vi "Auto_Targeting.vi"(1 "Acceptable Error (deg)":dbl, 2 "Auto Targeting Enabled?":bool) -> ()   [LabVIEW 2020]
uses:
  <vilib>/Rock Robotics/WPI/ThirdParty/REV Robotics/REVLib/Typedef/Spark MAX Control Type.ctl
  <vilib>/Rock Robotics/WPI/Utilities/WPI_GetSetVariantRefNum.vi
  Global Sensor Reads.vi
  Global Shooter Speed.vi
  <vilib>/Rock Robotics/WPI/RobotDrive/WPI_RobotDriveArcadeDrive_Standard(NoSaturation).vi
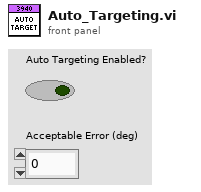
[diagram p1: front panel]
types:
  T1 = typedef "WPI_RobotDriveDevRef.ctl" = cluster{"DevStatus":errorcluster, "Motors[]":T2[], "Square Inputs":bool, "Max Output":dbl}
  T2 = typedef "WPI_MotorControlDeviceRef.ctl" = cluster{"DeviceStatus":errorcluster, "Type":T3, "PWM":cluster{"PWM Channel":T4, "DeadBand":T5}, "CAN":cluster{"Device Number":u8, "SetOutput VI Ref":variant, "GetOutput VI Ref":variant, "Enable VI Ref":variant, "Disable VI Ref":variant, "Data":variant}, "Invert":bool, "DIO PWM":cluster{"PWM \"Enable\" Channel":T4, "DIOChannel":T6, "PWM Rate":dbl}}
  T3 = typedef "WPI_MotorControlType.ctl" = enum16{"PWM", "CAN", "DIO PWM"}
  T4 = typedef "FPGA_DIOPWMChannel.ctl" = enum8{"PWM 0", "PWM 1", "PWM 2", "PWM 3", "PWM 4", "PWM 5", "PWM 6", "PWM 7", "PWM 8", "PWM 9", "PWM MXP 0", "PWM MXP 1", "PWM MXP 2", "PWM MXP 3", "PWM MXP 4", "PWM MXP 5", "PWM MXP 6", "PWM MXP 7", "PWM MXP 8", "PWM MXP 9", "Invalid"}
  T5 = typedef "WPI_PWMDeadband.ctl" = cluster{"Name":string, "maxPositivePwm":i32, "minPositivePwm":i32, "centerPwm":i32, "maxNegativePwm":i32, "minNegativePwm":i32, "angularRange":u16}
  T6 = typedef "FPGA_DIOChannel.ctl" = enum8{"DIO 0", "DIO 1", "DIO 2", "DIO 3", "DIO 4", "DIO 5", "DIO 6", "DIO 7", "DIO 8", "DIO 9", "DIO MXP 0", "DIO MXP 1", "DIO MXP 2", "DIO MXP 3", "DIO MXP 4", "DIO MXP 5", "DIO MXP 6", "DIO MXP 7", "DIO MXP 8", "DIO MXP 9", "DIO MXP 10", "DIO MXP 11", "DIO MXP 12", "DIO MXP 13", "DIO MXP 14", "DIO MXP 15", "SPI Port CS1", "SPI Port CS2", "SPI Port CS3", "SPI Port MISO", "SPI Port MOSI", "Invalid"}
  T7 = typedef "Spark MAX Control Type.ctl" = enum16{"Percent VBus", "Voltage", "Velocity", "Position", "Smart Motion", "Current", "Smart Velocity"}
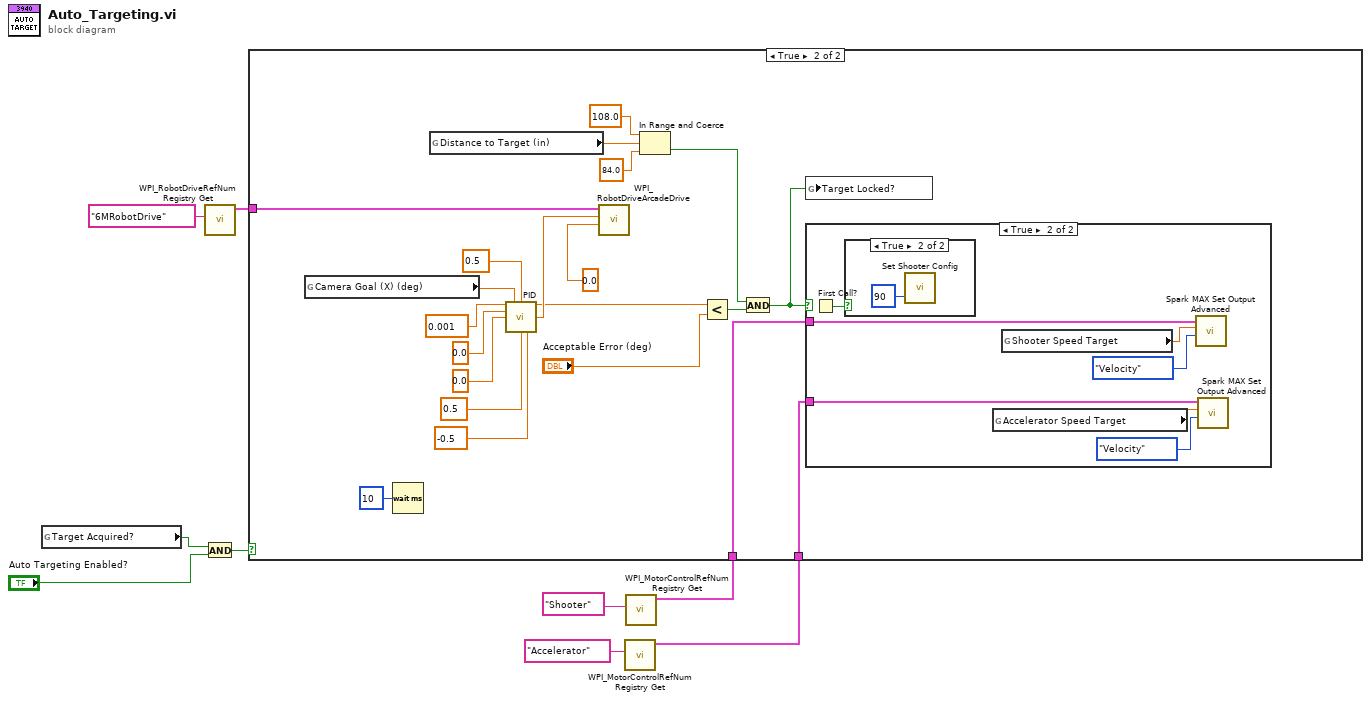
[diagram p0: block diagram]
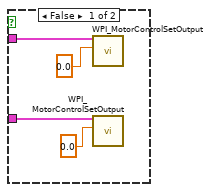
[diagram p3: hidden frame]
diagram:
  n1 = global read "Global Sensor Reads.vi" "Target Acquired?"() -> (w8:bool)
  n2 = call <vilib>:"WPI_RobotDriveRefNum Registry Get.vi"("refnum name"="6MRobotDrive") -> ("RobotDriveDevRef"=w4:T1)  [unwired: 9 in, 1 out]
  n3 = And(x=w8, y="Auto Targeting Enabled?") -> (x .and. y?=w9:bool)
  n4 = call <vilib>:"WPI_MotorControlRefNum Registry Get.vi"("refnum name"="Accelerator") -> ("MotorControlDevRef"=w2:T2)  [unwired: 9 in, 1 out]
  n5 = call <vilib>:"WPI_MotorControlRefNum Registry Get.vi"("refnum name"="Shooter") -> ("MotorControlDevRef"=w3:T2)  [unwired: 9 in, 1 out]
  n6 = case shown="True" w9 {
    tunnel: w4 -> [_ w30]
    tunnel: w3 -> [_ w29]
    tunnel: w2 -> [_ w28]
    frame False {
    }
    frame True {
      n7 = global read "Global Sensor Reads.vi" "Camera Goal (X) (deg)"() -> (w27:dbl)
      n8 = Wait (ms)(milliseconds to wait=u32 10) -> ()  [unwired: 1 out]
      n9 = global read "Global Sensor Reads.vi" "Distance to Target (in)"() -> (w15:dbl)
      n10 = call "PID.vi"("Kp"=0.001, "Process Variable"=w27, "Goal"=0.5, "Ki"=0.0, "Kd"=0.0, "Max Ouput"=0.5, "Min Output"=-0.5) -> ("Current Error"=w17:dbl, "Command"=w20:dbl)  [unwired: 6 in, 1 out]
      n11 = call-poly <vilib>:"WPI_RobotDriveArcadeDrive.vi"("Y axis value"=0.0, "X axis value"=w20, "RobotDriveDevRef"=w30) -> ()  [unwired: 6 in, 3 out]
      n12 = In Range and Coerce(upper limit=108.0, x=w15, lower limit=84.0) -> (In Range?=w11:bool)  [unwired: 1 out]
      n13 = Less?(x=w17, y="Acceptable Error (deg)") -> (x < y?=w12:bool)
      n14 = And(x=w11, y=w12) -> (x .and. y?=w10:bool)
      n15 = global write "Global Sensor Reads.vi" "Target Locked?"(w10) -> ()
      n16 = case shown="True" w10 {
        tunnel: w29 -> [w32 w36]
        tunnel: w28 -> [w31 w35]
        frame False {
          n17 = call <vilib>:"WPI_MotorControlSetOutput.vi"("Output"=0.0, "MotorControlDevRef"=w32) -> ()  [unwired: 7 in, 3 out]
          n18 = call <vilib>:"WPI_MotorControlSetOutput.vi"("Output"=0.0, "MotorControlDevRef"=w31) -> ()  [unwired: 7 in, 3 out]
        }
        frame True {
          n19 = First Call?() -> (First Call?: T/F=w41:bool)
          n20 = case shown="True" w41 {
            frame False {
            }
            frame True {
              n21 = call "Set Shooter Config.vi"("POV Joystick Input"=90) -> ()  [unwired: 3 in]
            }
          }
          n22 = global read "Global Shooter Speed.vi" "Accelerator Speed Target"() -> (w38:dbl)
          n23 = global read "Global Shooter Speed.vi" "Shooter Speed Target"() -> (w40:dbl)
          n24 = call <vilib>:"Spark MAX Set Output Advanced.vi"("Control Mode"=Spark_MAX_Control_Type."Velocity", "Setpoint"=w40, "MotorControlDevRef"=w36) -> ()  [unwired: 7 in, 2 out]
          n25 = call <vilib>:"Spark MAX Set Output Advanced.vi"("Control Mode"=Spark_MAX_Control_Type."Velocity", "Setpoint"=w38, "MotorControlDevRef"=w35) -> ()  [unwired: 7 in, 2 out]
        }
      }
    }
  }
